vi "Jacobian_f.vi"(8 "Alpha_r":dbl, 9 "Alpha_c":dbl, 10 "Sample Interval (sec)":dbl, 11 "Input State":T1) -> (3 "J_f":T2)   [LabVIEW 2019]
uses:
  <vilib>/Analysis/Matrix/Datatypes/RealMatrix.ctl
  <vilib>/Analysis/Matrix/NI_Matrix.lvlib
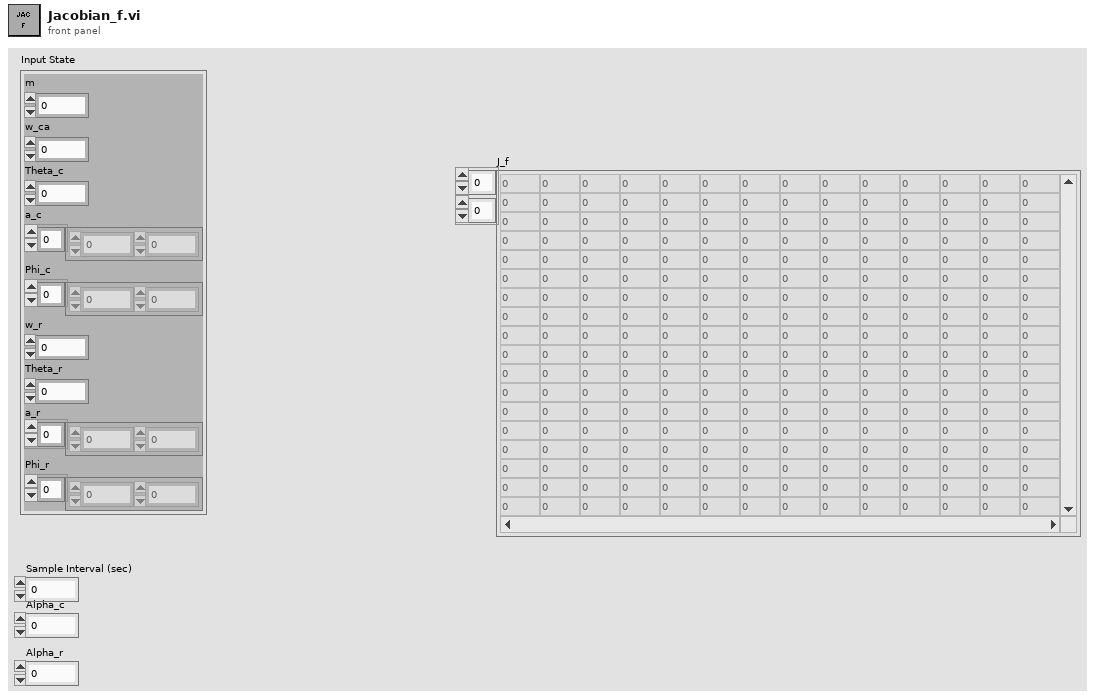
[diagram p1: front panel]
types:
  T1 = cluster{"m":dbl, "w_ca":dbl, "Theta_c":dbl, "a_c":dbl[], "Phi_c":dbl[], "w_r":dbl, "Theta_r":dbl, "a_r":dbl[], "Phi_r":dbl[]}
  T2 = typedef "NI_Matrix.lvlib/RealMatrix.ctl" = dbl[][]
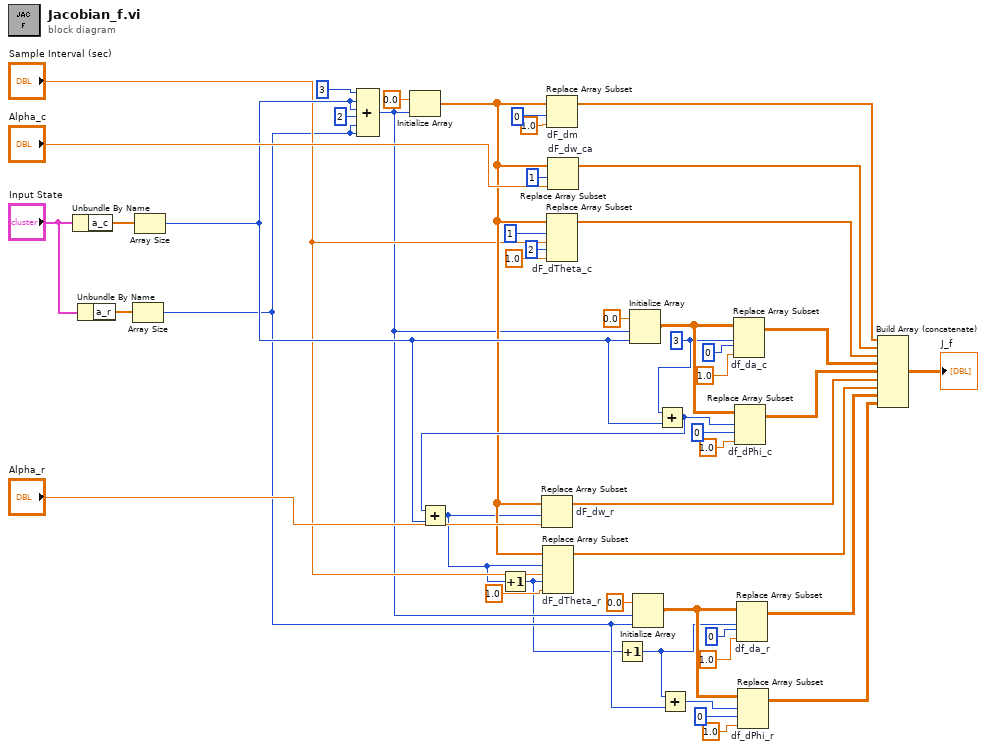
[diagram p0: block diagram]
diagram:
  w32 = 3 ("disabled index (row)")
  n1 = Unbundle By Name("Input State") -> ("a_c"=w1:dbl[])
  n2 = Unbundle By Name("Input State") -> ("a_r"=w3:dbl[])
  n3 = Array Size(array=w3) -> (size(s)=w13:i32)
  n4 = Array Size(array=w1) -> (size(s)=w29:i32)
  n5 = Compound Arithmetic op=ADD(3, w29, w29, 2 ("value"), w13, w13) -> (w14:i32)
  n6 = Initialize Array(0.0 ("element"), w14) -> (w23:dbl[])
  n7 = Replace Array Subset "dF_dm"(array=w23, new element=1.0 ("new element/subarray"), index=0) -> (w28:dbl[])
  n8 = Replace Array Subset "dF_dTheta_c"(array=w23, new element #1="Sample Interval (sec)", index #1=1 ("index"), new element #2=1.0 ("new element/subarray"), index #2=2 ("index")) -> (w6:dbl[])
  n9 = Replace Array Subset "dF_dw_ca"(array=w23, new element="Alpha_c", index=1) -> (w27:dbl[])
  n10 = Initialize Array(0.0 ("element"), w14, w29) -> (w33:dbl[][])
  n11 = Initialize Array(0.0 ("element"), w14, w13) -> (w20:dbl[][])
  n12 = Add(x=w32, y=w29) -> (x+y=w30:i32)
  n13 = Add(x=w30, y=w29) -> (x+y=w5:i32)
  n14 = Increment(x=w5) -> (x+1=w12:i32)
  n15 = Replace Array Subset "dF_dw_r"(array=w23, new element="Alpha_r", index=w5) -> (w7:dbl[])
  n16 = Replace Array Subset "dF_dTheta_r"(array=w23, new element #1="Sample Interval (sec)", index #1=w5, new element #2=1.0 ("new element/subarray"), index #2=w12) -> (w8:dbl[])
  n17 = Increment(x=w12) -> (x+1=w11:i32)
  n18 = Add(x=w11, y=w13) -> (x+y=w21:i32)
  n19 = Replace Array Subset "df_da_c"(array=w33, new element=1.0 ("new diagonal/fill element"), index (row)=w32, index (col)=0 ("disabled index (row)")) -> (w26:T2)
  n20 = Replace Array Subset "df_dPhi_c"(array=w33, new element=1.0 ("new diagonal/fill element"), index (row)=w30, index (col)=0 ("disabled index (row)")) -> (w25:T2)
  n21 = Replace Array Subset "df_da_r"(array=w20, new element=1.0 ("new diagonal/fill element"), index (row)=w11, index (col)=0 ("disabled index (row)")) -> (w9:T2)
  n22 = Replace Array Subset "df_dPhi_r"(array=w20, new element=1.0 ("new diagonal/fill element"), index (row)=w21, index (col)=0 ("disabled index (row)")) -> (w10:T2)
  n23 = Build Array (concatenate)(w28, w27, w6, w26, w25, w7, w8, w9, w10) -> (→"J_f":T2)
